vi "FTW-Inbox-Core-ConstructMessageRouter.vi"(0 "Actor Identity":string, 11 "error in":errorcluster) -> (1 "Incoming Message Registration":refnum<event-registration>, 3 "Message Pipe":refnum<queue>, 4 "Resolved Actor Identity":string, 6 "ActorStatus":T1, 8 "Incoming Message Notifier":refnum<user-event>, 15 "error out":errorcluster)   [LabVIEW 2015]
uses:
  core/type/FTW-Type-JSON.ctl
panel:
  # "Inputs"
  # "Outputs"
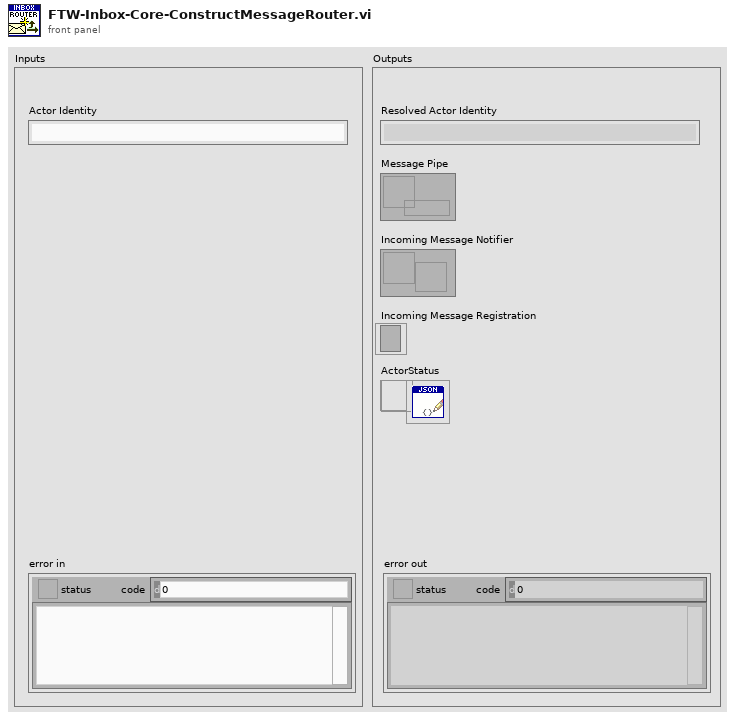
[diagram p1: front panel]
types:
  T1 = typedef "FTW-Type-JSON.ctl" = refnum<data-value>
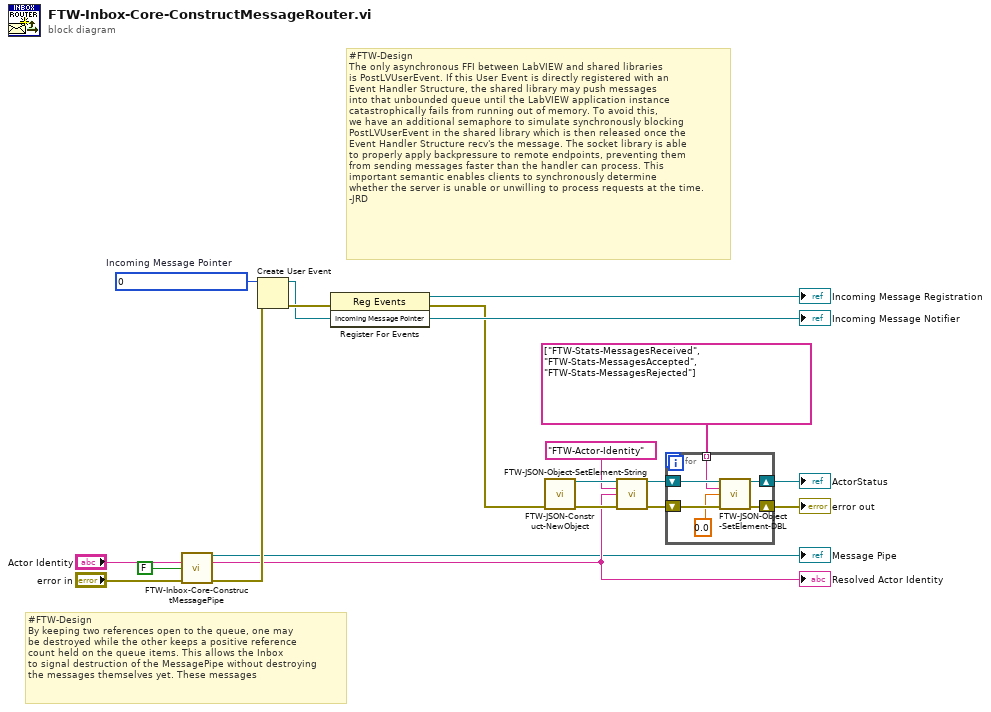
[diagram p0: block diagram]
diagram:
  w16 = i64 0  # Incoming Message Pointer
  # "#FTW-Design\nThe only asynchronous FFI between LabVIEW and shared libraries\nis PostLVUserEvent. If this User Event is directly registered with an\nEvent Handler Structure, the shared library may push messages\ninto that unbounded queue until the LabVIEW application instance\ncatastrophically fails from running out of memory. To avoid this,\nwe have an additional semaphore to simulate synchronously blocking\nPostLVUserEvent in the shared library which is then released once the\nEvent Handler Structure recv's the message. The socket library is able\nto properly apply backpressure to remote endpoints, preventing them\nfrom sending messages faster than the handler can process. This\nimportant semantic enables clients to synchronously determine\nwhether the server is unable or unwilling to process requests at the time.\n-JRD"
  # "#FTW-Design\nBy keeping two references open to the queue, one may\nbe destroyed while the other keeps a positive reference\ncount held on the queue items. This allows the Inbox\nto signal destruction of the MessagePipe without destroying\nthe messages themselves yet. These messages"
  n1 = call "FTW-Inbox-Core-ConstructMessagePipe.vi"("Actor Identity (empty to create unnamed actor)"="Actor Identity", "Is Primary?"=FALSE, "error in"="error in") -> ("Message Pipe"=→"Message Pipe":refnum<queue>, "Resolved Actor Identity"=w4:string, "error out"=w18:errorcluster)  [unwired: 10 in]
  "Resolved Actor Identity" <- w4
  n2 = Create User Event(user event datatype=w16, error in=w18) -> (user event=w7:refnum<user-event>, error out=w19:errorcluster)
  "Incoming Message Notifier" <- w7
  n3 = register-events(error in=w19, w7) -> (reference out=→"Incoming Message Registration":refnum<event-registration>, error out=w5:errorcluster)  [unwired: 1 in]
  n4 = call "FTW-JSON-Construct-NewObject.vi"("error in"=w5) -> ("JSON"=w13:T1, "error out"=w11:errorcluster)  [unwired: 13 in]
  n5 = call "FTW-JSON-Object-SetElement-String.vi"("JSON"=w13, "Key"="FTW-Actor-Identity", "Value"=w4, "error in"=w11) -> ("JSON out"=w9:T1, "error out"=w10:errorcluster)  [unwired: 10 in]
  n6 = for {
    shift-right: [w24] -> w1
    shift-left: w9 -> [w25]
    shift-right: [w22] -> w3
    shift-left: w10 -> [w23]
    tunnel: string[] ["FTW-Stats-MessagesReceived", "FTW-Stats-MessagesAccepted", "FTW-Stats-MessagesRejected"] -> [w21] mode=indexing
    n7 = call "FTW-JSON-Object-SetElement-DBL.vi"("JSON"=w25, "Key"=w21, "Value"=0.0, "error in"=w23) -> ("JSON out"=w24:T1, "error out"=w22:errorcluster)  [unwired: 10 in]
  }
  "error out" <- w3
  "ActorStatus" <- w1
